vi "Wind_Turbine_Control.vi"(3 "Mode":T5=enum."Run VI", 5 "Traverse line In":T2={"Start X"=0.0, "Start Y"=0.0, "Start Z"=0.0, "End X"=0.0, "End Y"=0.0, "End Z"=0.0, "No. of pts."=0, "Spacing"=enum."Linear", "Filename"=path "", "Tunnel Speed"=0.0, "Averaging time (min)"=0.0, "Extra Commands"="0.02 ; 1.0", "Carrier_1 Q (l/min)"=0.0, "Carrier_2 Q (l/min)"=0.0, "Trace Gas Concentration (%)"=0.0, "Specific Arguments"="Wind_Turbine_Control.vi; 600", "Comments"="", "Row No"=0, "Row Type Selector"=enum."Move Traverse Only", "Completion time"="", "Row Duration (mins)"=0.0, "No. of Valid pts."=0, "Meas Setup File"=""} {"Carrier_2 Q (l/min)" format="%#.2f"; "Row Duration (mins)" format="%#.1f"; "Row No" min=0; "Trace Gas Concentration (%)" min=0.0 format="%#_4f"; "Carrier_1 Q (l/min)" format="%#.2f"; "Tunnel Speed" format="%#.2f"; "Start X" format="%#.2f"; "Start Y" format="%#.2f"; "Start Z" format="%#.2f"; "End X" format="%#.2f"; "End Y" format="%#.2f"; "End Z" format="%#.2f"; "Averaging time (min)" min=0.0 format="%#.2f"}) -> (0 "Error Message":string, 1 "Status":T1, 2 "Traverse line Out":T2={"Start X"=0.0, "Start Y"=0.0, "Start Z"=0.0, "End X"=0.0, "End Y"=0.0, "End Z"=0.0, "No. of pts."=0, "Spacing"=enum."Linear", "Filename"=path "", "Tunnel Speed"=0.0, "Averaging time (min)"=0.0, "Extra Commands"="0.035 ; 0.1", "Carrier_1 Q (l/min)"=0.0, "Carrier_2 Q (l/min)"=0.0, "Trace Gas Concentration (%)"=0.0, "Specific Arguments"="Wind_Turbine_Control.vi; 600", "Comments"="", "Row No"=0, "Row Type Selector"=enum."Move Traverse Only", "Completion time"="", "Row Duration (mins)"=0.0, "No. of Valid pts."=0, "Meas Setup File"=""} {"Carrier_2 Q (l/min)" format="%#.2f"; "Row Duration (mins)" format="%#.1f"; "Row No" min=0; "Trace Gas Concentration (%)" min=0.0 format="%#_4f"; "Carrier_1 Q (l/min)" format="%#.2f"; "Tunnel Speed" format="%#.2f"; "Start X" format="%#.2f"; "Start Y" format="%#.2f"; "Start Z" format="%#.2f"; "End X" format="%#.2f"; "End Y" format="%#.2f"; "End Z" format="%#.2f"; "Averaging time (min)" min=0.0 format="%#.2f"})   [LabVIEW 2016]
uses:
  Gen Trav/Traverse_cluster.ctl
  Gen Trav/Spacing.ctl
  Controls/Multi_run_mode.ctl
  Controls/User_Specific_mode.ctl
  Gen Trav/Multi_Run_Status.ctl
panel:
  # "X           Y            Z"
  # "Start"
  # "End"
  # "X           Y            Z"
  # "Start"
  # "End"
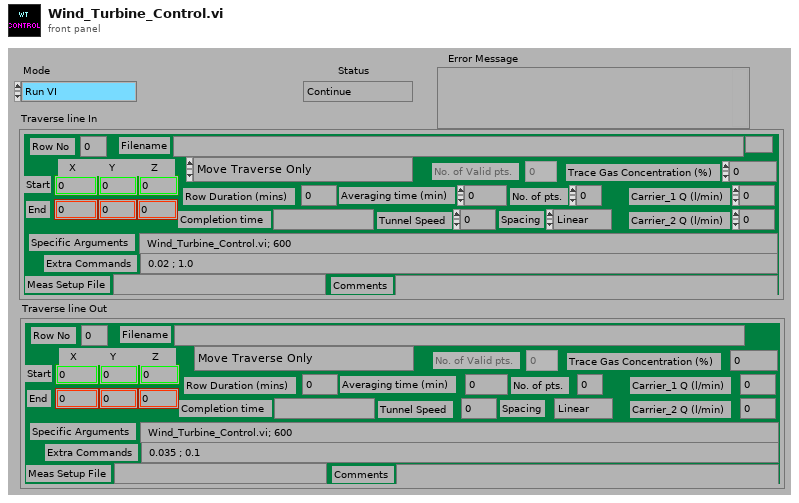
[diagram p1: front panel]
types:
  T1 = typedef "Multi_Run_Status.ctl" = enum16{"Continue", "Continue with Error", "Jump to Next Point", "Jump to Next Row", "Jump To Fall Back", "Terminate Run"}
  T2 = typedef "Traverse_cluster.ctl" = cluster{"Start X":sgl, "Start Y":sgl, "Start Z":sgl, "End X":sgl, "End Y":sgl, "End Z":sgl, "No. of pts.":i32, "Spacing":T3, "Filename":path, "Tunnel Speed":dbl, "Averaging time (min)":dbl, "Extra Commands":string, "Carrier_1 Q (l/min)":dbl, "Carrier_2 Q (l/min)":dbl, "Trace Gas Concentration (%)":dbl, "Specific Arguments":string, "Comments":string, "Row No":i32, "Row Type Selector":T4, "Completion time":string, "Row Duration (mins)":dbl, "No. of Valid pts.":i32, "Meas Setup File":string}
  T3 = typedef "Spacing.ctl" = enum16{"Linear", "Log", "Gauss", "Specified", "N/A"}
  T4 = typedef "Multi_run_mode.ctl" = enum16{"Move Traverse Only", "Set Tunnel Speed Only", "Set Source Only", "Set Measurement Conditions", "Single Measurement", "Vertical Profile", "Lateral Profile", "Longitudinal Profile", "Explore Volume", "Multi-Axis Profile", "Auto Calibrate", "Meas Fast FID Bkgnd", "Check Beam Power", "Scanning Valve Measurement", "Run VI Named:", "Set ADAM Ch", "Wait (minutes)", "Send Message", "Synchronize With:", "Fall Back to this Row", "Turn Off Row Repeating", "Blank Row", "Traverse 3D Volume"}
  T5 = typedef "User_Specific_mode.ctl" = enum16{"Check VI only", "Run VI"}
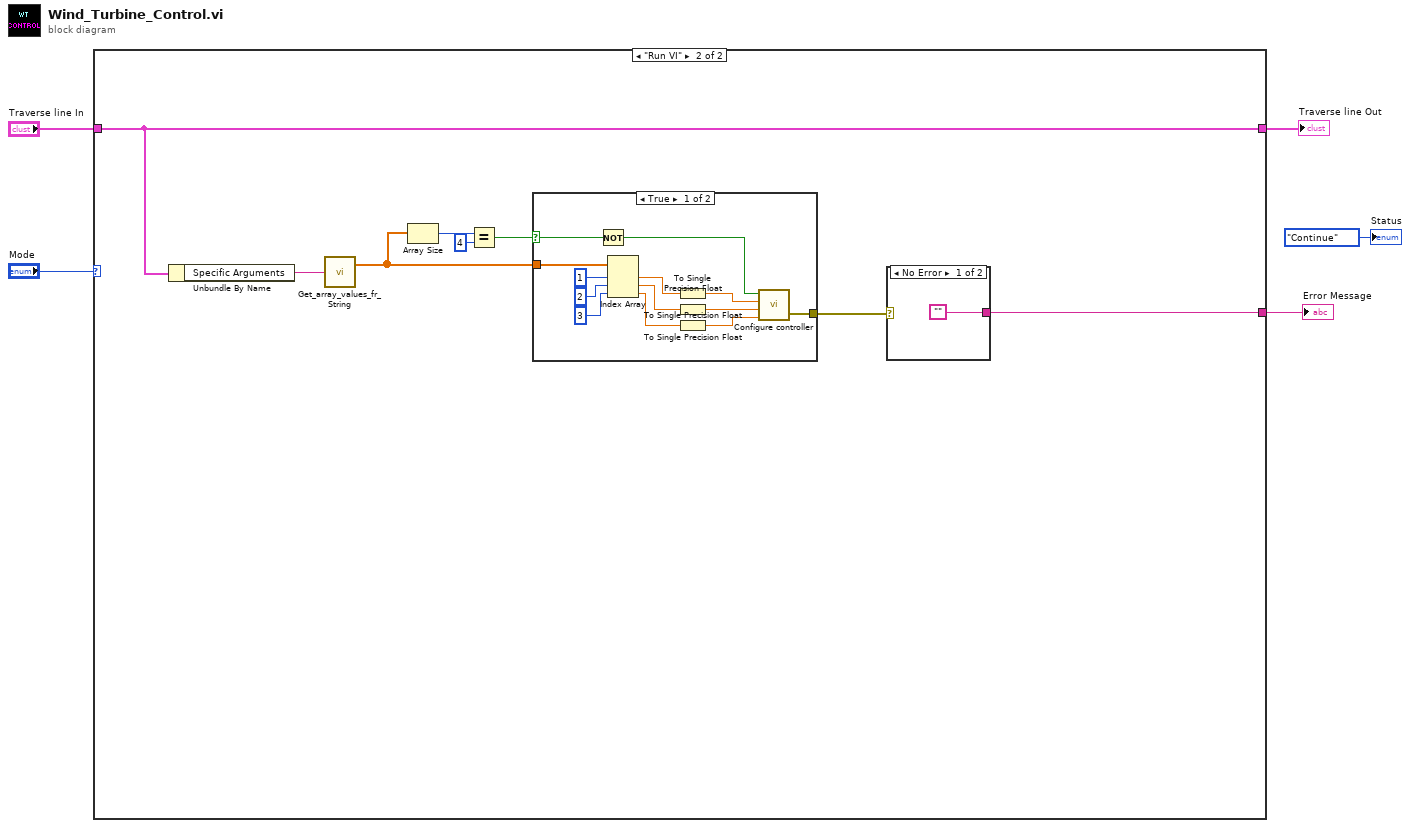
[diagram p0: block diagram]
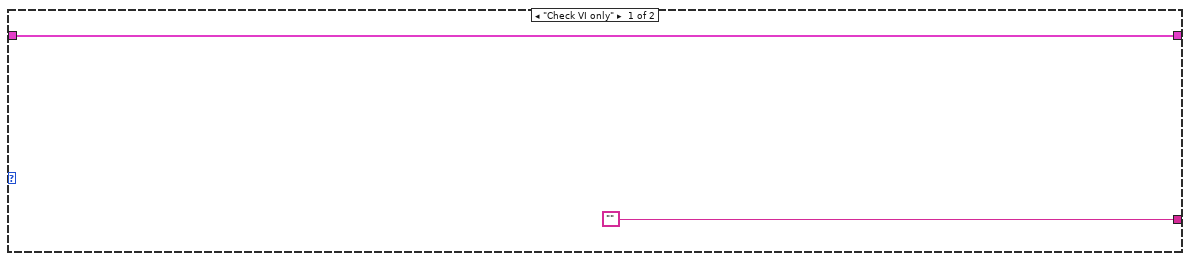
[diagram p2: hidden frame]
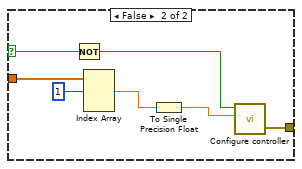
[diagram p3: hidden frame]
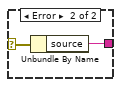
[diagram p4: hidden frame]
diagram:
  n1 = case shown="\"Run VI\"" "Mode" {
    tunnel: "Traverse line In" -> [w7 w15]
    tunnel: [w7 w15] -> w3
    tunnel: ["" w13] -> w2
    frame "Check VI only" {
    }
    frame "Run VI" {
      n2 = Unbundle By Name(w15) -> ("Specific Arguments"=w14:string)
      n3 = call "Get_array_values_fr_String.vi"("String Value"=w14) -> ("Numeric Array"=w11:dbl[])  [unwired: 1 out]
      n4 = Array Size(array=w11) -> (size(s)=w10:i32)
      n5 = Equal?(x=w10, y=4) -> (x = y?=w8:bool)
      n6 = case shown="True" w8 {
        selector: w8 -> [w23 w30]
        tunnel: [w27 w34] -> w12
        tunnel: w11 -> [w24 w31]
        frame True {
          n7 = Not(x=w23) -> (.not. x?=w16:bool)
          n8 = Index Array(array=w24, index #1=1 ("index"), index #2=2 ("index"), index #3=3 ("index")) -> (element #1=w26:dbl, element #2=w21:dbl, element #3=w22:dbl)
          n9 = To Single Precision Float(number=w26) -> (single precision float=w25:sgl)
          n10 = To Single Precision Float(number=w21) -> (single precision float=w20:sgl)
          n11 = To Single Precision Float(number=w22) -> (single precision float=w19:sgl)
          n12 = call "Configure controller.vi"("Ti (s)"=w19, "Kp"=w20, "RPM"=w25, "Set RPM only (else full config.)"=w16) -> ("error out"=w27:errorcluster)  [unwired: 1 in]
        }
        frame False {
          n13 = Not(x=w30) -> (.not. x?=w29:bool)
          n14 = Index Array(array=w31, index #1=1 ("index")) -> (element #1=w33:dbl)  [unwired: 2 in, 2 out]
          n15 = To Single Precision Float(number=w33) -> (single precision float=w32:sgl)
          n16 = call "Configure controller.vi"("RPM"=w32, "Set RPM only (else full config.)"=w29) -> ("error out"=w34:errorcluster)  [unwired: 3 in]
        }
      }
      n17 = case shown="No Error" w12 {
        selector: w12 -> [_ w37]
        tunnel: ["" w38] -> w13
        frame No Error {
        }
        frame Error {
          n18 = Unbundle By Name(w37) -> ("source"=w38:string)
        }
      }
    }
  }
  "Traverse line Out" <- w3
  "Error Message" <- w2
  "Status" <- Multi_Run_Status."Continue" ("Status")
